vi "GetDeviceName.vi"(7 "PortQuantity":i32, 10 "Input":string[](array[string])) -> (2 "Output":string[](array[string]))   [LabVIEW 2020]
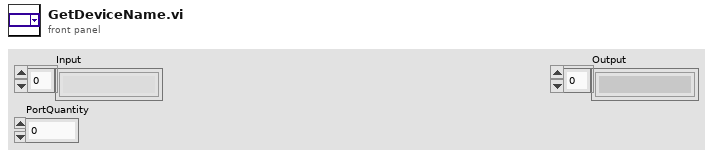
[diagram p1: front panel]
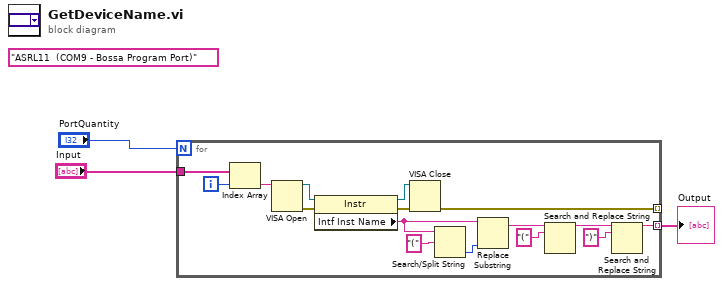
[diagram p0: block diagram]
diagram:
  (unwired) "ASRL11  (COM9 - Bossa Program Port)" ("string")
  n1 = for {
    N: "PortQuantity" -> [_]
    tunnel: "Input" -> [w14]
    tunnel: [w6] -> w2 mode=indexing
    tunnel: [w4] -> _ mode=indexing
    i -> [w19]
    n2 = Index Array(array=w14, index=w19) -> (element=w5:string)
    n3 = VISA Open(VISA resource name=w5) -> (VISA resource name=w18:refnum<visa-resource-name>, error out=w17:errorcluster)  [unwired: 4 in]
    n4 = property class="Instr"(reference=w18, error in=w17) -> (reference out=w15:refnum<visa-resource-name>, error out=w16:errorcluster, "Intf Inst Name"=w7:string)
    n5 = VISA Close(VISA resource name=w15, error in (no error)=w16) -> (error out=w4:errorcluster)
    n6 = Search/Split String(string=w7, search string/char (-)="(") -> (offset of match=w9:i32)  [unwired: 1 in, 2 out]
    n7 = Replace Substring(2:w9, 5:w7) -> (1:w10:string)  [unwired: 2 in, 1 out]
    n8 = Search and Replace String(input string=w10, search string="(") -> (result string=w13:string)  [unwired: 6 in, 3 out]
    n9 = Search and Replace String(input string=w13, search string=")") -> (result string=w6:string)  [unwired: 6 in, 3 out]
  }
  "Output" <- w2
